vi "exception to json error cluster.vi"(8 "exception":T1 {"code" format="%.0x"}) -> (0 "error in":errorcluster)   [LabVIEW 2013]
uses:
  exception.ctl
  const sourcename.vi
  <vilib>/addons/JSON API/Variant JSON/Variant to JSON.vi
  <vilib>/addons/JSON API/JSON Value/Get as JSON string (pretty).vi
  exception.lvlib
  <vilib>/addons/JSON API/Get Polymorphic/JSON GetSet.lvlib
  <vilib>/addons/JSON API/JSON Value/JSON Value.lvclass
  <vilib>/addons/JSON API/Variant JSON/Variant JSON.lvlib
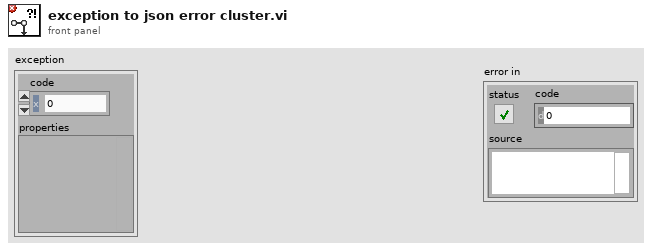
[diagram p1: front panel]
types:
  T1 = typedef "exception.lvlib/exception.ctl" = cluster{"code":i32, "properties":variant}
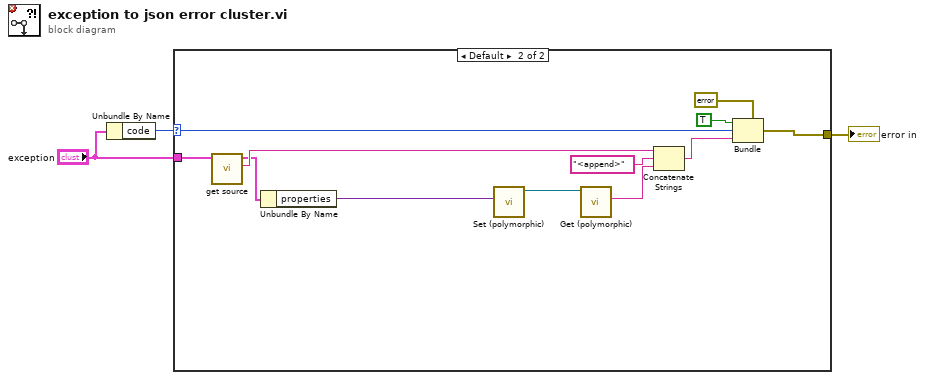
[diagram p0: block diagram]
diagram:
  n1 = Unbundle By Name("exception") -> ("code"=w2:i32)
  n2 = case shown="Default" w2 {
    selector: w2 -> [_ w14]
    tunnel: [_ w15] -> w3
    tunnel: "exception" -> [_ w13]
    frame 0 {
    }
    frame Default {
      n3 = call "get source.vi"("exception in"=w13) -> ("source"=w11:string, "exception out"=w10:T1)  [unwired: 9 in]
      n4 = Unbundle By Name(w10) -> ("properties"=w6:variant)
      n5 = call-poly <vilib>:"Set (polymorphic).vi"("Variant"=w6) -> ("JSON Value out"=w7:refnum<class "JSON Value.lvclass">)  [unwired: 9 in, 1 out]
      n6 = call-poly <vilib>:"Get (polymorphic).vi"("JSON Value in"=w7) -> ("String"=w5:string)  [unwired: 9 in, 1 out]
      n7 = Concatenate Strings(w11, "<append>" ("string"), w5) -> (w8:string)
      n8 = Bundle(cluster=errorcluster {"status"=FALSE, "code"=0, "source"=""} ("error in 2"), "status"=TRUE, "code"=w14, "source"=w8) -> (w15:errorcluster)
    }
  }
  "error in" <- w3
